vi "Acquire.vi"(0 "Cluster":T3={"Camera.lvclass"=refnum, "InClusTiming 2"={"Pixelclock"=24, "Exposure"=46.39115, "ExposureTimeBase"=2, "Framerate"=14.99615, "TriggerMode"=0}, "ROI"={"PosX"=0, "PosY"=0, "Width"=0, "Height"=0}, "File Path Control"=path "", "mirror.lvclass"=refnum} {"InClusTiming 2"."TriggerMode" items=["Auto", "Software", "External sequence start ", "External exposure control"]; "InClusTiming 2"."ExposureTimeBase" items=["nanoseconds", "microseconds", "milliseconds"]; "InClusTiming 2"."Pixelclock" min=1 max=400 step=1 scale=0.05915..400.0 scale format="%#.3g"; "InClusTiming 2"."Framerate" min=0.05915 max=2000.0 step=1.0 scale=0.05915..100.0 scale format="%#.3g"; "InClusTiming 2"."Exposure" min=0.05915 max=2000.0 step=1.0 scale=0.05915..100.0 scale format="%#.3g"}, 7 "clustPointagFin":T1, 11 "error in (no error)":errorcluster) -> (4 "Cluster 2":T3={"Camera.lvclass"=refnum, "InClusTiming 2"={"Pixelclock"=24, "Exposure"=46.39115, "ExposureTimeBase"=2, "Framerate"=14.99615, "TriggerMode"=0}, "ROI"={"PosX"=0, "PosY"=0, "Width"=0, "Height"=0}, "File Path Control"=path "", "mirror.lvclass"=refnum} {"InClusTiming 2"."TriggerMode" items=["Auto", "Software", "External sequence start ", "External exposure control"]; "InClusTiming 2"."ExposureTimeBase" items=["nanoseconds", "microseconds", "milliseconds"]; "InClusTiming 2"."Pixelclock" min=1 max=400 step=1 scale=0.05915..400.0 scale format="%#.3g"; "InClusTiming 2"."Framerate" min=0.05915 max=2000.0 step=1.0 scale=0.05915..100.0 scale format="%#.3g"; "InClusTiming 2"."Exposure" min=0.05915 max=2000.0 step=1.0 scale=0.05915..100.0 scale format="%#.3g"}, 6 "clustBufferNumber":cluster{"processedFPS":dbl, "Buffer Number":u32}, 8 "clustPointagFin":T1, 15 "error out":errorcluster)   [LabVIEW 2020, in "Acquisition.lvlib"]
doc: "Perform the acquisition. Replace the contents of this diagram with calls to acquisition hardware."
uses:
  Acquisition.lvlib
  HardwareConfiguration.ctl
  CLASS/Image Acquisition Class/Camera.lvclass
  MIRROR/mirror.lvclass
  SETTING/clustOA.ctl
  <vilib>/Analysis/Matrix/Datatypes/RealMatrix.ctl
  <vilib>/Analysis/Matrix/NI_Matrix.lvlib
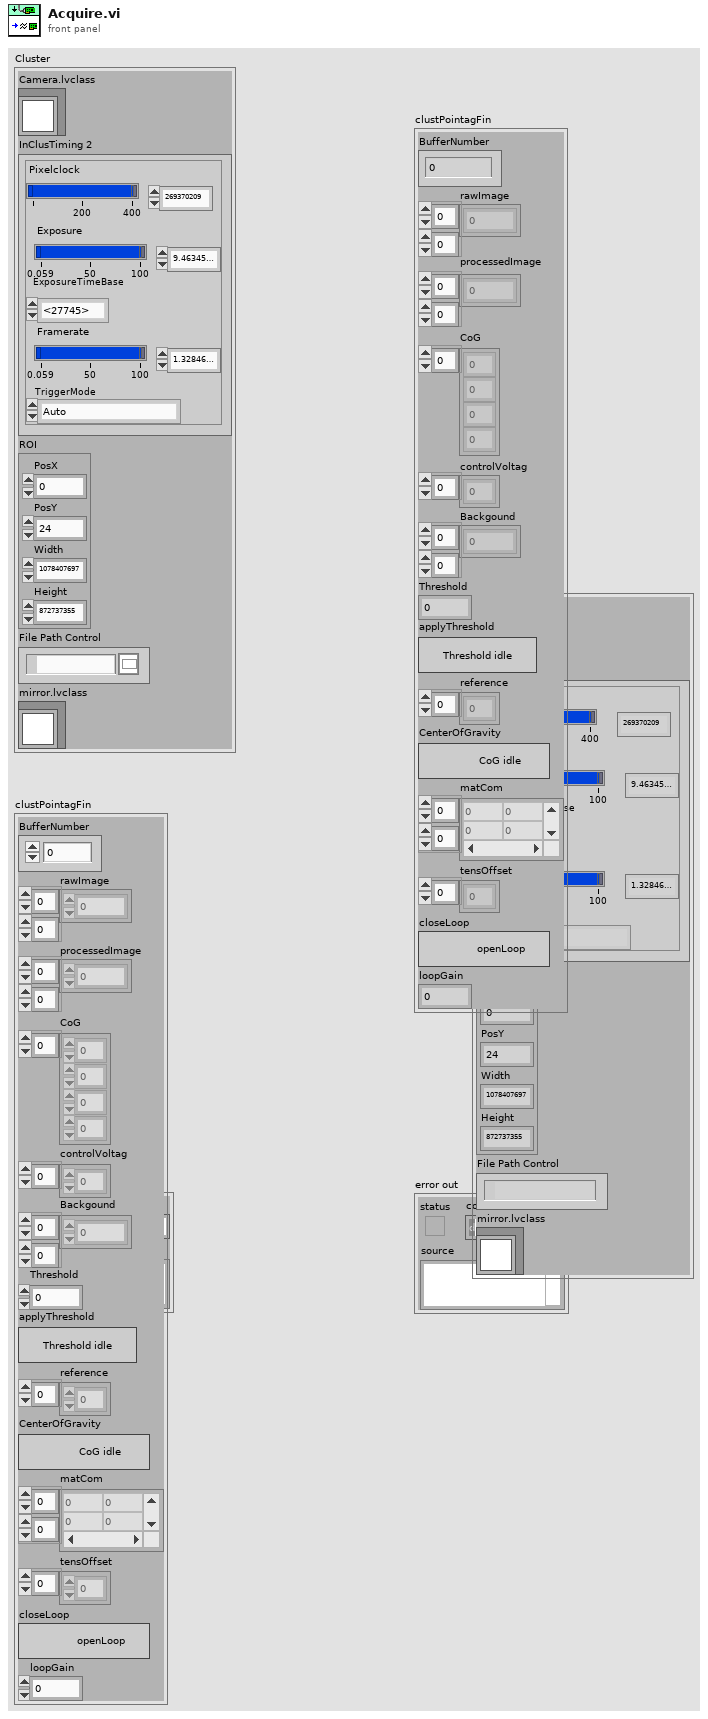
[diagram p1: front panel]
types:
  T1 = typedef "clustOA.ctl" = cluster{"BufferNumber":u32, "rawImage":u16[][], "processedImage":sgl[][], "CoG":dbl[], "controlVoltag":dbl[], "Backgound":sgl[][], "Threshold":dbl, "applyThreshold":bool, "reference":dbl[], "CenterOfGravity":bool, "matCom":T2, "tensOffset":dbl[], "closeLoop":bool, "loopGain":dbl}
  T2 = typedef "NI_Matrix.lvlib/RealMatrix.ctl" = dbl[][]
  T3 = typedef "Acquisition.lvlib/HardwareConfiguration.ctl" = cluster{"Camera.lvclass":refnum<class "Camera.lvclass">, "InClusTiming 2":cluster{"Pixelclock":i32, "Exposure":dbl, "ExposureTimeBase":u16, "Framerate":dbl, "TriggerMode":u16}, "ROI":cluster{"PosX":i32, "PosY":i32, "Width":i32, "Height":i32}, "File Path Control":path, "mirror.lvclass":refnum<class "mirror.lvclass">}
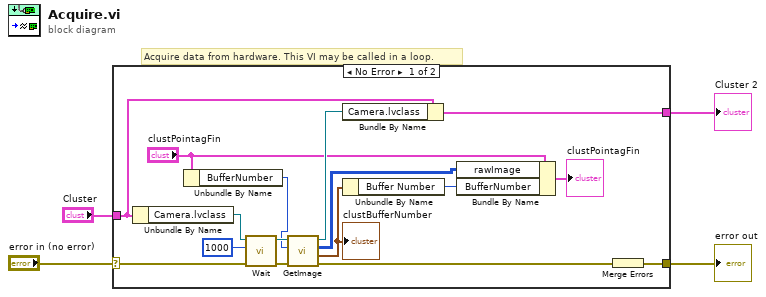
[diagram p0: block diagram]
diagram:
  # "Acquire data from hardware. This VI may be called in a loop."
  n1 = case shown="No Error" "error in (no error)" {
    selector: "error in (no error)" -> [w11 w21]
    tunnel: [w20 w21] -> w3
    tunnel: "Cluster" -> [w18 w22]
    tunnel: [w17 w22] -> w2
    frame No Error {
      n2 = Unbundle By Name(w18) -> ("Camera.lvclass"=w14:refnum<class "Camera.lvclass">)
      n3 = Unbundle By Name("clustPointagFin") -> ("BufferNumber"=w5:u32)
      n4 = call-dynamic "Wait.vi"("error in (no error)"=w11, "Timeout"=1000, "Camera in"=w14) -> ("error out"=w12:errorcluster, "Camera out"=w13:refnum<class "Camera.lvclass">)  [unwired: 7 in]
      n5 = call-dynamic "GetImage.vi"("error in (no error)"=w12, "inBufferNumber"=w5, "Image Acquisition in"=w13) -> ("error out"=w19:errorcluster, "Cluster"=w8:cluster{"processedFPS":dbl, "Buffer Number":u32}, "Image Reference"=w10:u16[][], "Image Acquisition out"=w16:refnum<class "Camera.lvclass">)  [unwired: 5 in]
      "clustBufferNumber" <- w8
      n6 = Bundle By Name(cluster=w18, "Camera.lvclass"=w16) -> (w17:T3)
      n7 = Unbundle By Name(w8) -> ("Buffer Number"=w7:u32)
      n8 = Bundle By Name(cluster="clustPointagFin", "rawImage"=w10, "BufferNumber"=w7) -> (→"clustPointagFin":T1)
      n9 = Merge Errors(w19) -> (w20:errorcluster)
    }
    frame Error {
    }
  }
  "error out" <- w3
  "Cluster 2" <- w2
